vi "OSIPI OPCUA Server Tag Version.vi"(11 "Main Queue Cluster":T4) -> ()   [LabVIEW 2018]
uses:
  <vilib>/OPCUA/controls/NodeId.ctl
  <vilib>/OPCUA/controls/OPC UA Variable Node Refnum.ctl
  <vilib>/OPCUA/controls/OPC UA Server Refnum.ctl
  Drag and Drop/State Cluster.ctl
  support/Message Queue/Message Cluster.ctl
  Drag and Drop/Thumbnail Cluster.ctl
  Drag and Drop/Object Cluster.ctl
  <vilib>/Utility/miscctls.llb/LVRectTypeDef.ctl
  Drag and Drop/Object Type Enum.ctl
  <vilib>/Utility/miscctls.llb/LVPositionTypeDef.ctl
  Config Module/Controls/Main Config Cluster.ctl
  OPC Module Config.ctl
  Scale Module Folder/Measure Instrument/State Enum.ctl
  <vilib>/Utility/miscctls.llb/LVPoint32TypeDef.ctl
  OPC Settings.ctl
  Variable Data Cluster.ctl
  <vilib>/OPCUA/controls/OPC UA StatusCode.ctl
  <vilib>/OPCUA/controls/Subscription ID.ctl
  <vilib>/OPCUA/controls/OPC UA Client Refnum.ctl
  <vilib>/OPCUA/controls/Subscription Data Change.ctl
  <vilib>/OPCUA/controls/Data Type.ctl
  OPC Tag Data.ctl
  Feed Module/Controls/Feed Module Config Cluster.ctl
  Feed Module/Controls/Feed Module Settings Cluster.ctl
  Ismatec ISM 831C/Controls/Ismatech ISM831C Settings Cluster.ctl
  Masterflex 7550-30/Controls/Settings Cluster.ctl
  Mettler Toledo/Controls/Settings Cluster.ctl
  Bronkhorst M13 Flow Meter/Settings Cluster.ctl
  Measure Instrument/PID 2 Parameters Cluster.ctl
  Measure Instrument/PID Input Enum.ctl
  Measure Instrument/PID 2 Output Enum.ctl
  Tacmina QI/Tacmina QI DAQ Setting.ctl
  KNF Pump/Settings Cluster plus SIMDOS.ctl
  ASIA Pump/Pump Settings.ctl
  VICI M50 Party Mode/Settings Cluster.ctl
  FLOM Pump/Settings Cluster.ctl
  SSI PR Class/SSI PR or LD Settings Cluster.ctl
  Masterflex 75211/Masterflex 75211 DAQ Setting.ctl
  SSI PR Class/SSI P40 Settings Cluster.ctl
  Ismatec 78001/Ismatec 4083.ctl
  Bronkhorst M14 Flow Meter/Settings Cluster.ctl
  TT Module/Controls/TT Module Config Cluster.ctl
  Tag VIs/Numeric Alarm Settings Cluster.ctl
  Acquisition/Hardware Configuration.ctl
  Acquisition/Task Cluster.ctl
  PT Module/Controls/PT Module Config Cluster.ctl
  Scale Module Folder/Feed Module/Controls/Scale Module Config Cluster.ctl
  Scale Module Folder/Feed Module/Controls/Scale Module Settings Cluster.ctl
  Pump Module Folder/Pump Module Config Cluster.ctl
  Pump Module Folder/Pump Module Settings Cluster.ctl
  LabJack Module/Controls/U3 Module Config Cluster.ctl
  Decoration Module/Decoration Module Config Cluster.ctl
  Flow Module Folder/Feed Module/Controls/Flow Module Config Cluster.ctl
  Flow Module Folder/Feed Module/Controls/Flow Module Settings Cluster.ctl
  TCU Module/TCU Module Folder/TCU Module Config Cluster.ctl
  TCU Module/TCU Module Folder/TCU Module Settings Cluster.ctl
  TCU Module/TCU Module Folder/Measure Instrument/Output Devices.ctl
  Huber TCU/Huber Settings.ctl
  Lauda Integral XT-150 TCU/Lauda Settings.ctl
  Julabo Type 1 TCU/Julabo Type 1 TCU Folder/Julabo FP-50 Settings.ctl
  Huber Unistat 410 TCU/Huber Unistat 410 RS485 Settings.ctl
  D-O Module Folder/Not Sure Where this is Used.ctl
  Sequencing/Squence Control.ctl
  D-O Module Folder/D-O Module Config Cluster.ctl
  D-O Module Folder/Valve Clusters.ctl
  D-O Module Folder/D-O Module Settings Cluster.ctl
  D-O Module Folder/D-O Device Settings Cluster.ctl
  VICI Electronic Actuator/VICI Electronic Actuator Settings.ctl
  Pressure Regulator Control Module/Pressure Regulator/Controls/4-20mA Module Config Cluster.ctl
  Pressure Regulator Control Module/Pressure Regulator/Controls/4-20mA Module Settings Cluster.ctl
  Pressure Transmitter/Pressure Transmitter Device Settings.ctl
  Pressure Reg Module/Pressure Regulator Device Settings.ctl
  Sonicator Module Folder/Feed Module/Controls/Sonicator Module Config Cluster.ctl
  Sonicator Module Folder/Feed Module/Controls/Sonicator Module Settings Cluster.ctl
  Sonic Systems P100/Sonic Systems P100 Settings.ctl
  Agitator Module Folder/Feed Module/Controls/Agitator Module Config Cluster.ctl
  Agitator Module Folder/Feed Module/Controls/Agitator Module Settings Cluster.ctl
  <vilib>/OPCUA/controls/Supported Security Policies.ctl
  Main/Main Queue Cluster.ctl
  Tag VIs/Tag FGV Operation Enum.ctl
  <vilib>/OPCUA/server/Write Double.vi
  <vilib>/regexp/Match Regular Expression.xnode
  <vilib>/OPCUA/NI OPC UA Server.lvlib
  Shared Variables/Dynamic Shared Variables.lvlib
  support/Message Queue/Message Queue.lvlib
  support/Message Queue/Enqueue Message (Single).vi
  TT Module/TT Module.lvlib
  Masterflex 7550-30/Masterflex 7550-30.lvlib
  Ismatec ISM 831C/Ismatec ISM 831C.lvlib
  Tacmina QI/Tacmina QI.lvlib
  KNF Pump/KNF SIMDOS.lvlib
  VICI M50 Party Mode/VICI M6 M50 Party Mode.lvlib
  FLOM Pump/FLOM Pump.lvlib
  ASIA Pump.lvlib
  Mettler Toledo/Mettler Toledo.lvlib
  Bronkhorst M13 Flow Meter/Bronkhorst M13 Flow Meter.lvlib
  SSI PR Class/SSI PR or LD Pump.lvlib
  Feed Module/Feed Module.lvlib
  DAQ/DAQ.lvlib
  PT Module/PT Module.lvlib
  Scale Module Folder/Scale Module.lvlib
  Pump Module Folder/Pump Module.lvlib
  LabJack Module/U3 Module.lvlib
  Flow Module Folder/Flow Module.lvlib
  Huber TCU/Huber Ministat 230 TCU.lvlib
  Lauda Integral XT-150 TCU/Lauda TCU.lvlib
  Julabo Type 1 TCU/Julabo Type 1 TCU Folder/Julabo Type FP-50 TCU.lvlib
  TCU Module/TCU Module Folder/TCU Module.lvlib
  Sequencing/Sequencing Library.lvlib
  D-O Module Folder/D-O Module.lvlib
  D-O Module Folder/DIO Valve/VICI Electronic Actuator.lvlib
  Pressure Transmitter/Pressure Transmitter Library.lvlib
  Pressure Reg Module/Pressure Regulator Library.lvlib
  Pressure Regulator Control Module/Pressure Regulator/4-20mA Module.lvlib
  OPC UA.lvlib
  Scale Module Folder/Measure Instrument/Scale Module Engine.lvlib
  Config Module/Config Module.lvlib
  Drag and Drop/Drag and Drop.lvlib
  Masterflex 75211/Masterflex 75211.lvlib
  SSI PR Class/SSI P40 Pump.lvlib
  Huber Unistat 410 TCU/Huber Unistat 410 TCU.lvlib
  Ismatec 78001/Ismatec 4308.lvlib
  Bronkhorst M14 Flow Meter/Bronkhorst M14 Flow Meter.lvlib
  Sonicator Module Folder/Sonicator Module.lvlib
  Sonic Systems P100/Sonic Systems P100.lvlib
  Agitator Module Folder/Agitator Module.lvlib
panel:
  out "Array 4":T3(array[cluster])
  in  "?":T5 {"Main Config"."PR Module Configs"."Settings"."PID 2 Parameters"."output range"."output low" format="%.2f"; "Main Config"."PR Module Configs"."Settings"."PID 2 Parameters"."output range"."output high" min=0.0 max=100.0 format="%.2f"; "Main Config"."PR Module Configs"."Settings"."PID 2 Parameters"."PID gains"."derivative time (Td, min)" format="%.3f"; "Main Config"."PR Module Configs"."Settings"."PID 2 Parameters"."PID gains"."integral time (Ti, min)" format="%.3f"; "Main Config"."PR Module Configs"."Settings"."PID 2 Parameters"."PID gains"."proportional gain (Kc)" format="%.3f"; "Main Config"."Steps"."Control" items=["Pump %", "Setpoint"]; "Main Config"."TCU Module Configs"."Settings"."Huber Unistat 410 Settings"."Address" min=0 max=99 format="%02.0f"; "Main Config"."TCU Module Configs"."Settings"."Julabo FP-50 Settings"."Pump Power" min=0 max=8 step=1; "Main Config"."TCU Module Configs"."Settings"."Lauda Settings"."Pump Power" min=0 max=8 step=1; "Main Config"."Flow Module Configs"."Settings"."Bronkhorst M14 Settings"."Smoothing Steps" min=1 step=1; "Main Config"."Flow Module Configs"."Settings"."Bronkhorst M13 Settings"."Smoothing Steps" min=1 step=1; "Main Config"."Pump Module Configs"."Settings"."Ismatech 3 Channel Settings"."Channel Number" min=0 max=3; "Main Config"."Pump Module Configs"."Settings"."Ismatech 3 Channel Settings"."Pump Number" min=1; "Main Config"."Pump Module Configs"."Settings"."ASIA Pump C"."channel" min=0 max=1 step=1; "Main Config"."Pump Module Configs"."Settings"."Masterflex"."Pump Number" min=1.0 max=20.0 step=1.0; "Main Config"."Pump Module Configs"."Settings"."Ismatech"."Pump Number" min=1.0 max=20.0 step=1.0; "Main Config"."Feed Module Configs"."Settings"."Bronkhorst M14 Settings"."Smoothing Steps" min=1 step=1; "Main Config"."Feed Module Configs"."Settings"."Ismatech 3 Channel Settings"."Channel Number" min=0 max=3; "Main Config"."Feed Module Configs"."Settings"."Ismatech 3 Channel Settings"."Pump Number" min=1; "Main Config"."Feed Module Configs"."Settings"."output range"."output low" min=0.0 max=100.0 format="%.2f"; "Main Config"."Feed Module Configs"."Settings"."output range"."output high" format="%.2f"; "Main Config"."Feed Module Configs"."Settings"."PID 2 Parameters"."PID gains"."derivative time (Td, min)" format="%.3f"; "Main Config"."Feed Module Configs"."Settings"."PID 2 Parameters"."PID gains"."integral time (Ti, min)" format="%.3f"; "Main Config"."Feed Module Configs"."Settings"."PID 2 Parameters"."PID gains"."proportional gain (Kc)" format="%.3f"; "Main Config"."Feed Module Configs"."Settings"."Bronkhorst M13 Flow Meter"."Smoothing Steps" min=1 step=1; "Main Config"."Feed Module Configs"."Settings"."ASIA Pump C"."channel" min=0 max=1 step=1; "Main Config"."Feed Module Configs"."Settings"."Ismatech"."Pump Number" min=1.0 max=20.0 step=1.0; "Main Config"."Feed Module Configs"."Settings"."Masterflex"."Pump Number" min=1.0 max=20.0 step=1.0}
  in  "supported security policies (None)":T76={"None"=TRUE, "Sign with Basic128Rsa15"=TRUE, "Sign and Encrypt with Basic128Rsa15"=TRUE, "Sign with Basic256"=TRUE, "Sign and Encrypt with Basic256"=TRUE}
  out "Tag Values":dbl[](array[numeric])
  out "Tag Names":string[](array[string])
  out "Array":T3(array[cluster])
  out "OPC UA server refnum out":T77
  out "Array 2":T17[](array[typedef]) items=["Good"=0, "Good_SubscriptionTransferred"=2949120, "Good_CompletesAsynchronously"=3014656, "Good_Overload"=3080192, "Good_Clamped"=3145728, "Good_LocalOverride"=9830400, "Good_EntryInserted"=10616832, "Good_EntryReplaced"=10682368, "Good_NoData"=10813440, "Good_MoreData"=10878976, "Good_CommunicationEvent"=10944512, "Good_ShutdownEvent"=11010048, "Good_CallAgain"=11075584, "Good_NonCriticalTimeout"=11141120, "Good_ResultsMayBeIncomplete"=12189696, "Good_DataIgnored"=14221312, "Uncertain"=1073741824, "Uncertain_ReferenceOutOfServer"=1080819712, "Uncertain_NoCommunicationLastUsableValue"=1083113472, "Uncertain_LastUsableValue"=1083179008, "Uncertain_SubstituteValue"=1083244544, "Uncertain_InitialValue"=1083310080, "Uncertain_SensorNotAccurate"=1083375616, "Uncertain_EngineeringUnitsExceeded"=1083441152, "Uncertain_SubNormal"=1083506688, "Uncertain_DataSubNormal"=1084489728, "Uncertain_ReferenceNotDeleted"=1086062592, "Uncertain_NotAllNodesAvailable"=1086324736, "Bad"=2147483648, "Bad_UnexpectedError"=2147549184, "Bad_InternalError"=2147614720, "Bad_OutOfMemory"=2147680256, "Bad_ResourceUnavailable"=2147745792, "Bad_CommunicationError"=2147811328, "Bad_EncodingError"=2147876864, "Bad_DecodingError"=2147942400, "Bad_EncodingLimitsExceeded"=2148007936, "Bad_UnknownResponse"=2148073472, "Bad_Timeout"=2148139008, "Bad_ServiceUnsupported"=2148204544, "Bad_Shutdown"=2148270080, "Bad_ServerNotConnected"=2148335616, "Bad_ServerHalted"=2148401152, "Bad_NothingToDo"=2148466688, "Bad_TooManyOperations"=2148532224, "Bad_DataTypeIdUnknown"=2148597760, "Bad_CertificateInvalid"=2148663296, "Bad_SecurityChecksFailed"=2148728832, "Bad_CertificateTimeInvalid"=2148794368, "Bad_CertificateIssuerTimeInvalid"=2148859904, "Bad_CertificateHostNameInvalid"=2148925440, "Bad_CertificateUriInvalid"=2148990976, "Bad_CertificateUseNotAllowed"=2149056512, "Bad_CertificateIssuerUseNotAllowed"=2149122048, "Bad_CertificateUntrusted"=2149187584, "Bad_CertificateRevocationUnknown"=2149253120, "Bad_CertificateIssuerRevocationUnknown"=2149318656, "Bad_CertificateRevoked"=2149384192, "Bad_CertificateIssuerRevoked"=2149449728, "Bad_UserAccessDenied"=2149515264, "Bad_IdentityTokenInvalid"=2149580800, "Bad_IdentityTokenRejected"=2149646336, "Bad_SecureChannelIdInvalid"=2149711872, "Bad_InvalidTimestamp"=2149777408, "Bad_NonceInvalid"=2149842944, "Bad_SessionIdInvalid"=2149908480, "Bad_SessionClosed"=2149974016, "Bad_SessionNotActivated"=2150039552, "Bad_SubscriptionIdInvalid"=2150105088, "Bad_RequestHeaderInvalid"=2150236160, "Bad_TimestampsToReturnInvalid"=2150301696, "Bad_RequestCancelledByClient"=2150367232, "Bad_NoCommunication"=2150694912, "Bad_WaitingForInitialData"=2150760448, "Bad_NodeIdInvalid"=2150825984, "Bad_NodeIdUnknown"=2150891520, "Bad_AttributeIdInvalid"=2150957056, "Bad_IndexRangeInvalid"=2151022592, "Bad_IndexRangeNoData"=2151088128, "Bad_DataEncodingInvalid"=2151153664, "Bad_DataEncodingUnsupported"=2151219200, "Bad_NotReadable"=2151284736, "Bad_NotWritable"=2151350272, "Bad_OutOfRange"=2151415808, "Bad_NotSupported"=2151481344, "Bad_NotFound"=2151546880, "Bad_ObjectDeleted"=2151612416, "Bad_NotImplemented"=2151677952, "Bad_MonitoringModeInvalid"=2151743488, "Bad_MonitoredItemIdInvalid"=2151809024, "Bad_MonitoredItemFilterInvalid"=2151874560, "Bad_MonitoredItemFilterUnsupported"=2151940096, "Bad_FilterNotAllowed"=2152005632, "Bad_StructureMissing"=2152071168, "Bad_EventFilterInvalid"=2152136704, "Bad_ContentFilterInvalid"=2152202240, "Bad_FilterOperandInvalid"=2152267776, "Bad_ContinuationPointInvalid"=2152333312, "Bad_NoContinuationPoints"=2152398848, "Bad_ReferenceTypeIdInvalid"=2152464384, "Bad_BrowseDirectionInvalid"=2152529920, "Bad_NodeNotInView"=2152595456, "Bad_ServerUriInvalid"=2152660992, "Bad_ServerNameMissing"=2152726528, "Bad_DiscoveryUrlMissing"=2152792064, "Bad_SempahoreFileMissing"=2152857600, "Bad_RequestTypeInvalid"=2152923136, "Bad_SecurityModeRejected"=2152988672, "Bad_SecurityPolicyRejected"=2153054208, "Bad_TooManySessions"=2153119744, "Bad_UserSignatureInvalid"=2153185280, "Bad_ApplicationSignatureInvalid"=2153250816, "Bad_NoValidCertificates"=2153316352, "Bad_RequestCancelledByRequest"=2153381888, "Bad_ParentNodeIdInvalid"=2153447424, "Bad_ReferenceNotAllowed"=2153512960, "Bad_NodeIdRejected"=2153578496, "Bad_NodeIdExists"=2153644032, "Bad_NodeClassInvalid"=2153709568, "Bad_BrowseNameInvalid"=2153775104, "Bad_BrowseNameDuplicated"=2153840640, "Bad_NodeAttributesInvalid"=2153906176, "Bad_TypeDefinitionInvalid"=2153971712, "Bad_SourceNodeIdInvalid"=2154037248, "Bad_TargetNodeIdInvalid"=2154102784, "Bad_DuplicateReferenceNotAllowed"=2154168320, "Bad_InvalidSelfReference"=2154233856, "Bad_ReferenceLocalOnly"=2154299392, "Bad_NoDeleteRights"=2154364928, "Bad_ServerIndexInvalid"=2154430464, "Bad_ViewIdUnknown"=2154496000, "Bad_TooManyMatches"=2154627072, "Bad_QueryTooComplex"=2154692608, "Bad_NoMatch"=2154758144, "Bad_MaxAgeInvalid"=2154823680, "Bad_HistoryOperationInvalid"=2154889216, "Bad_HistoryOperationUnsupported"=2154954752, "Bad_WriteNotSupported"=2155020288, "Bad_TypeMismatch"=2155085824, "Bad_MethodInvalid"=2155151360, "Bad_ArgumentsMissing"=2155216896, "Bad_TooManySubscriptions"=2155282432, "Bad_TooManyPublishRequests"=2155347968, "Bad_NoSubscription"=2155413504, "Bad_SequenceNumberUnknown"=2155479040, "Bad_MessageNotAvailable"=2155544576, "Bad_InsufficientClientProfile"=2155610112, "Bad_TcpServerTooBusy"=2155675648, "Bad_TcpMessageTypeInvalid"=2155741184, "Bad_TcpSecureChannelUnknown"=2155806720, "Bad_TcpMessageTooLarge"=2155872256, "Bad_TcpNotEnoughResources"=2155937792, "Bad_TcpInternalError"=2156003328, "Bad_TcpEndpointUrlInvalid"=2156068864, "Bad_RequestInterrupted"=2156134400, "Bad_RequestTimeout"=2156199936, "Bad_SecureChannelClosed"=2156265472, "Bad_SecureChannelTokenUnknown"=2156331008, "Bad_SequenceNumberInvalid"=2156396544, "Bad_ConfigurationError"=2156462080, "Bad_NotConnected"=2156527616, "Bad_DeviceFailure"=2156593152, "Bad_SensorFailure"=2156658688, "Bad_OutOfService"=2156724224, "Bad_DeadbandFilterInvalid"=2156789760, "Bad_RefreshInProgress"=2157379584, "Bad_ConditionAlreadyDisabled"=2157445120, "Bad_ConditionDisabled"=2157510656, "Bad_EventIdUnknown"=2157576192, "Bad_NoData"=2157641728, "Bad_DataLost"=2157772800, "Bad_DataUnavailable"=2157838336, "Bad_EntryExists"=2157903872, "Bad_NoEntryExists"=2157969408, "Bad_TimestampNotSupported"=2158034944, "Bad_InvalidArgument"=2158690304, "Bad_ConnectionRejected"=2158755840, "Bad_Disconnect"=2158821376, "Bad_ConnectionClosed"=2158886912, "Bad_InvalidState"=2158952448, "Bad_EndOfStream"=2159017984, "Bad_NoDataAvailable"=2159083520, "Bad_WaitingForResponse"=2159149056, "Bad_OperationAbandoned"=2159214592, "Bad_ExpectedStreamToBlock"=2159280128, "Bad_WouldBlock"=2159345664, "Bad_SyntaxError"=2159411200, "Bad_MaxConnectionsReached"=2159476736, "Bad_RequestTooLarge"=2159542272, "Bad_ResponseTooLarge"=2159607808, "Bad_EventNotAcknowledgeable"=2159738880, "Bad_InvalidTimestampArgument"=2159869952, "Bad_ProtocolVersionUnsupported"=2159935488, "Bad_StateNotActive"=2160001024, "Bad_FilterOperatorInvalid"=2160132096, "Bad_FilterOperatorUnsupported"=2160197632, "Bad_FilterOperandCountMismatch"=2160263168, "Bad_FilterElementInvalid"=2160328704, "Bad_FilterLiteralInvalid"=2160394240, "Bad_IdentityChangeNotSupported"=2160459776, "Bad_NotTypeDefinition"=2160590848, "Bad_ViewTimestampInvalid"=2160656384, "Bad_ViewParameterMismatch"=2160721920, "Bad_ViewVersionInvalid"=2160787456, "Bad_ConditionAlreadyEnabled"=2160852992, "Bad_DialogNotActive"=2160918528, "Bad_DialogResponseInvalid"=2160984064, "Bad_ConditionBranchAlreadyAcked"=2161049600, "Bad_ConditionBranchAlreadyConfirmed"=2161115136, "Bad_ConditionAlreadyShelved"=2161180672, "Bad_ConditionNotShelved"=2161246208, "Bad_ShelvingTimeOutOfRange"=2161311744, "Bad_AggregateListMismatch"=2161377280, "Bad_AggregateNotSupported"=2161442816, "Bad_AggregateInvalidInputs"=2161508352, "Bad_BoundNotFound"=2161573888, "Bad_BoundNotSupported"=2161639424, "Bad_AggregateConfigurationRejected"=2161770496, "Bad_TooManyMonitoredItems"=2161836032]
  out "server endpoint URL":string
  in  "?":T5 {"Main Config"."PR Module Configs"."Settings"."PID 2 Parameters"."output range"."output low" format="%.2f"; "Main Config"."PR Module Configs"."Settings"."PID 2 Parameters"."output range"."output high" min=0.0 max=100.0 format="%.2f"; "Main Config"."PR Module Configs"."Settings"."PID 2 Parameters"."PID gains"."derivative time (Td, min)" format="%.3f"; "Main Config"."PR Module Configs"."Settings"."PID 2 Parameters"."PID gains"."integral time (Ti, min)" format="%.3f"; "Main Config"."PR Module Configs"."Settings"."PID 2 Parameters"."PID gains"."proportional gain (Kc)" format="%.3f"; "Main Config"."Steps"."Control" items=["Pump %", "Setpoint"]; "Main Config"."TCU Module Configs"."Settings"."Huber Unistat 410 Settings"."Address" min=0 max=99 format="%02.0f"; "Main Config"."TCU Module Configs"."Settings"."Julabo FP-50 Settings"."Pump Power" min=0 max=8 step=1; "Main Config"."TCU Module Configs"."Settings"."Lauda Settings"."Pump Power" min=0 max=8 step=1; "Main Config"."Flow Module Configs"."Settings"."Bronkhorst M14 Settings"."Smoothing Steps" min=1 step=1; "Main Config"."Flow Module Configs"."Settings"."Bronkhorst M13 Settings"."Smoothing Steps" min=1 step=1; "Main Config"."Pump Module Configs"."Settings"."Ismatech 3 Channel Settings"."Channel Number" min=0 max=3; "Main Config"."Pump Module Configs"."Settings"."Ismatech 3 Channel Settings"."Pump Number" min=1; "Main Config"."Pump Module Configs"."Settings"."ASIA Pump C"."channel" min=0 max=1 step=1; "Main Config"."Pump Module Configs"."Settings"."Masterflex"."Pump Number" min=1.0 max=20.0 step=1.0; "Main Config"."Pump Module Configs"."Settings"."Ismatech"."Pump Number" min=1.0 max=20.0 step=1.0; "Main Config"."Feed Module Configs"."Settings"."Bronkhorst M14 Settings"."Smoothing Steps" min=1 step=1; "Main Config"."Feed Module Configs"."Settings"."Ismatech 3 Channel Settings"."Channel Number" min=0 max=3; "Main Config"."Feed Module Configs"."Settings"."Ismatech 3 Channel Settings"."Pump Number" min=1; "Main Config"."Feed Module Configs"."Settings"."output range"."output low" min=0.0 max=100.0 format="%.2f"; "Main Config"."Feed Module Configs"."Settings"."output range"."output high" format="%.2f"; "Main Config"."Feed Module Configs"."Settings"."PID 2 Parameters"."PID gains"."derivative time (Td, min)" format="%.3f"; "Main Config"."Feed Module Configs"."Settings"."PID 2 Parameters"."PID gains"."integral time (Ti, min)" format="%.3f"; "Main Config"."Feed Module Configs"."Settings"."PID 2 Parameters"."PID gains"."proportional gain (Kc)" format="%.3f"; "Main Config"."Feed Module Configs"."Settings"."Bronkhorst M13 Flow Meter"."Smoothing Steps" min=1 step=1; "Main Config"."Feed Module Configs"."Settings"."ASIA Pump C"."channel" min=0 max=1 step=1; "Main Config"."Feed Module Configs"."Settings"."Ismatech"."Pump Number" min=1.0 max=20.0 step=1.0; "Main Config"."Feed Module Configs"."Settings"."Masterflex"."Pump Number" min=1.0 max=20.0 step=1.0}
  out "OPC UA server refnum out 3":T77
  out "Array 3":T3(array[cluster])
  # "Agitator Settings"
  # "Sonicator Settings"
  # "Instrument Settings"
  # "Instrument Settings"
  # "Output Instruments"
  # "Flow Meter Settings"
  # "Output Instruments"
  # "Scale Settings"
  # "Output Instruments"
  # "Input Instruments"
  # "Agitator Settings"
  # "Sonicator Settings"
  # "Instrument Settings"
  # "Instrument Settings"
  # "Output Instruments"
  # "Flow Meter Settings"
  # "Output Instruments"
  # "Scale Settings"
  # "Output Instruments"
  # "Input Instruments"
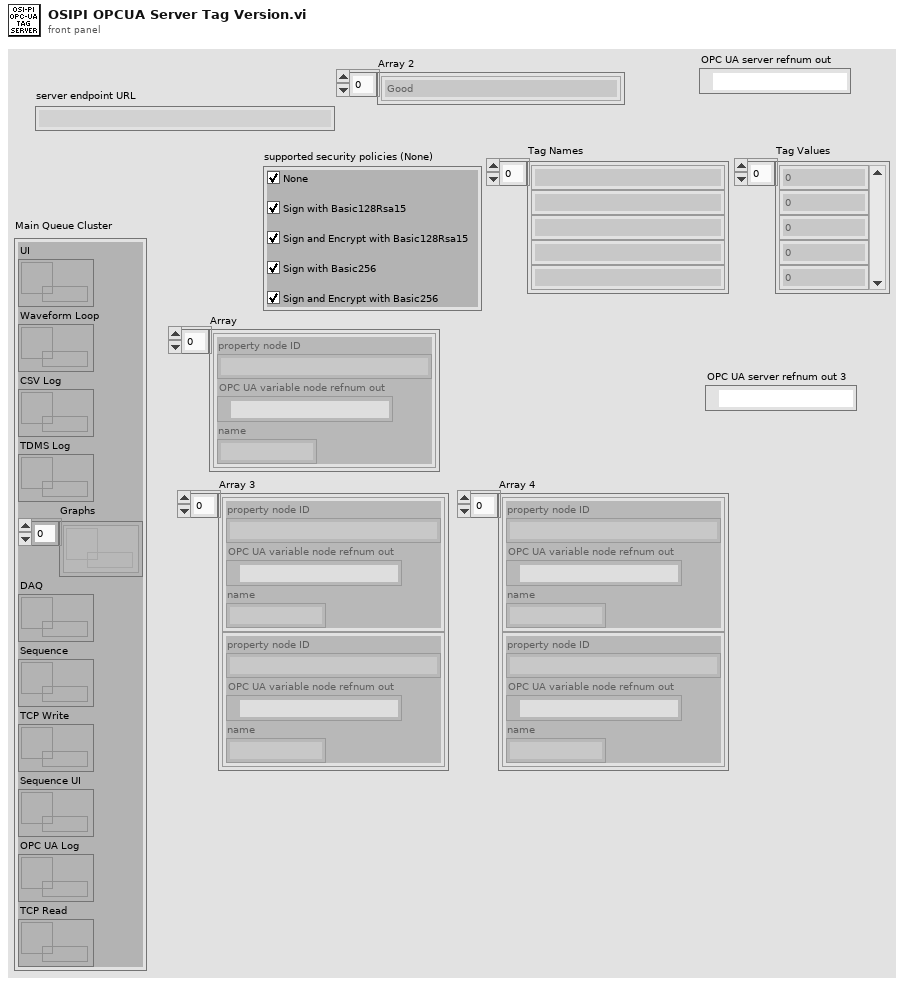
[diagram p1: front panel]
types:
  T1 = typedef "NodeId.ctl" = string
  T2 = typedef "OPC UA Variable Node Refnum.ctl" = refnum<k21>
  T3 = cluster{"property node ID":T1, "OPC UA variable node refnum out":T2, "name":string}[]
  T4 = typedef "Main Queue Cluster.ctl" = cluster{"UI":refnum<queue>, "Waveform Loop":refnum<queue>, "CSV Log":refnum<queue>, "TDMS Log":refnum<queue>, "Graphs":refnum<queue>[], "DAQ":refnum<queue>, "Sequence":refnum<queue>, "TCP Write":refnum<queue>, "Sequence UI":refnum<queue>, "OPC UA Log":refnum<queue>, "TCP Read":refnum<queue>}
  T5 = typedef "Drag and Drop.lvlib/State Cluster.ctl" = cluster{"VI refs":refnum<vi>[], "Queues":refnum<queue>[], "[Thumbnails]":T6[], "Drag Object Idx":i32, "[Objects]":T7[], "Active Object":i32, "Drop Offset":T10, "Process Name":string, "Main Config":T11, "Campaign Filepath":path, "Config Changed?":bool}
  T6 = typedef "Thumbnail Cluster.ctl" = cluster{"Path":path, "Rectangle":cluster{"left":i16, "top":i16, "right":i16, "bottom":i16}}
  T7 = typedef "Object Cluster.ctl" = cluster{"BMP Path":path, "Anchor Position":cluster{"X":i32, "Y":i32}, "Hot Spot":T8, "Type":T9, "Parameters":variant}
  T8 = typedef "LVRectTypeDef.ctl" = cluster{"Left":i16, "Top":i16, "Right":i16, "Bottom":i16}
  T9 = typedef "Object Type Enum.ctl" = enum16{"Icon", "Line", "Text", "Feed Module"}
  T10 = typedef "LVPositionTypeDef.ctl" = cluster{"Left":i32, "Top":i32}
  T11 = typedef "Config Module.lvlib/Main Config Cluster.ctl" = cluster{"Notebook":string, "OPC Module Configs":T12[], "Feed Module Configs":T21[], "Log File Path":path, "TT Module Configs":T40[], "DAQ Config":T42, "PT Module Configs":T44[], "Scale Module Configs":T45[], "Pump Module Configs":T47[], "U3 Module Configs":T49[], "Decoration Module Configs":T50[], "Flow Module Configs":T51[], "TCU Module Configs":T53[], "Steps":T60, "Abort":bool, "DO Module Configs":T62[], "PR Module Configs":T67[], "SC Module Configs":T71[], "AM Module Configs":T74[], "Cycle Period":dbl}
  T12 = typedef "OPC UA.lvlib/OPC Module Config.ctl" = cluster{"State":T13, "GUID":string, "Drop Coords":T14, "Configuration":T15, "First Iteration":bool, "Data":cluster{"Object Name":string, "Variable Array":T16[]}[], "Process Name":string, "Load Count":i32, "Log Started":bool, "subscription ID out":T18, "OPC UA client refnum out":T19, "Event Registration Refnum":refnum<event-registration>, "Start Time":timestamp, "Current Time":timestamp, "Tag Data":T20[]}
  T13 = typedef "Scale Module.lvlib/Scale Module Engine.lvlib/State Enum.ctl" = enum16{"Measuring", "Idle"}
  T14 = typedef "LVPoint32TypeDef.ctl" = cluster{"Horizontal":i32, "Vertical":i32}
  T15 = typedef "OPC UA.lvlib/OPC Settings.ctl" = cluster{"Cycle Period":dbl, "server endpoint URL":string, "security policy":cluster{"message mode":enum16{"None", "Sign", "Sign and Encrypt"}, "security":enum16{"Basic256", "Basic128Rsa15"}}, "Trust Any Server":bool}
  T16 = typedef "OPC UA.lvlib/Variable Data Cluster.ctl" = cluster{"node ID":T1, "browse name":string, "status":T17, "timestamp":timestamp, "value ":variant}
  T17 = typedef "OPC UA StatusCode.ctl" = u32
  T18 = typedef "Subscription ID.ctl" = u32
  T19 = typedef "OPC UA Client Refnum.ctl" = refnum<k21>
  T20 = typedef "OPC UA.lvlib/OPC Tag Data.ctl" = cluster{"Include this Device":bool, "Device Name":string, "OPC Tag Data":cluster{"Tag":string, "Value":variant, "Time Stamp":timestamp}[]}
  T21 = typedef "Feed Module.lvlib/Feed Module Config Cluster.ctl" = cluster{"GUID":string, "Drop Coords":T14, "Process Name":string, "Queue Name":string, "Settings":T22, "Settings Load Count":i32, "OP Load Count":i32}
  T22 = typedef "Feed Module.lvlib/Feed Module Settings Cluster.ctl" = cluster{"Cycle Period":dbl, "Ismatech":T23, "Masterflex":T24, "Mettler":T25, "Bronkhorst M13 Flow Meter":T26, "PID 2 Parameters":T27, "Manual Entry":dbl, "Auto?":bool, "output range":cluster{"output high":dbl, "output low":dbl}, "Tacmina Settings":T30, "KNF SIMDOS Settings":T31, "ASIA Pump C":T32, "VICI Settings":T33, "FLOM Settings":T34, "SSI PR/LD Settings":T35, "Masterflex 75211 Settings":T36, "SSI P40 Settings":T37, "Ismatech 3 Channel Settings":T38, "Bronkhorst M14 Settings":T39}
  T23 = typedef "Ismatec ISM 831C.lvlib/Ismatech ISM831C Settings Cluster.ctl" = cluster{"VISA resource name":refnum<visa-resource-name>, "Simulated?":bool, "Pump Number":dbl, "Reverse?":bool}
  T24 = typedef "Masterflex 7550-30.lvlib/Settings Cluster.ctl" = cluster{"VISA resource name":refnum<visa-resource-name>, "Simulated?":bool, "Pump Number":dbl, "Reverse?":bool}
  T25 = typedef "Mettler Toledo.lvlib/Settings Cluster.ctl" = cluster{"VISA resource name":refnum<visa-resource-name>, "Simulated?":bool}
  T26 = typedef "Bronkhorst M13 Flow Meter.lvlib/Settings Cluster.ctl" = cluster{"VISA resource name":refnum<visa-resource-name>, "Simulated?":bool, "Smoothing Steps":i32}
  T27 = typedef "PID 2 Parameters Cluster.ctl" = cluster{"Input Device":T28, "Output Device":T29, "Setpoint":dbl, "PID gains":cluster{"proportional gain (Kc)":dbl, "integral time (Ti, min)":dbl, "derivative time (Td, min)":dbl}}
  T28 = typedef "PID Input Enum.ctl" = enum16{"Default", "Bronkhorst M13", "Bronkhorst M14", "Scale Rate of Change"}
  T29 = typedef "PID 2 Output Enum.ctl" = enum16{"Default", "Ismatec ISM 4308", "Ismatec ISM 831C", "Masterflex 7550-30", "VICI", "Tacmina QI", "KNF SIMDOS", "ASIA Type C", "FLOM UI-22-11", "SSI PR/LD", "SSI P40", "Masterflex 75211-70"}
  T30 = typedef "Tacmina QI.lvlib/Tacmina QI DAQ Setting.ctl" = cluster{"Analog DAQ Task":refnum<k21>, "Digital DAQ Task":refnum<k21>}
  T31 = typedef "KNF SIMDOS.lvlib/Settings Cluster plus SIMDOS.ctl" = cluster{"VISA resource name":refnum<visa-resource-name>, "Simulated?":bool}
  T32 = typedef "ASIA Pump.lvlib/Pump Settings.ctl" = cluster{"ASIA Pump #":i32, "channel":i32, "Simulated":bool}
  T33 = typedef "VICI M6 M50 Party Mode.lvlib/Settings Cluster.ctl" = cluster{"VISA resource name":refnum<visa-resource-name>, "Simulated?":bool, "Pump Letter":string, "Reverse?":bool}
  T34 = typedef "FLOM Pump.lvlib/Settings Cluster.ctl" = cluster{"VISA resource name":refnum<visa-resource-name>, "Simulated?":bool, "Pump Number":dbl}
  T35 = typedef "SSI PR or LD Pump.lvlib/SSI PR or LD Settings Cluster.ctl" = cluster{"VISA resource name":refnum<visa-resource-name>, "Simulated?":bool}
  T36 = typedef "Masterflex 75211.lvlib/Masterflex 75211 DAQ Setting.ctl" = cluster{"Analog DAQ Task":refnum<k21>, "Digital DAQ Task":refnum<k21>}
  T37 = typedef "SSI P40 Pump.lvlib/SSI P40 Settings Cluster.ctl" = cluster{"VISA resource name":refnum<visa-resource-name>, "Simulated?":bool}
  T38 = typedef "Ismatec 4308.lvlib/Ismatec 4083.ctl" = cluster{"VISA resource name":refnum<visa-resource-name>, "Pump Number":i16, "Channel Number":i16, "Simulated?":bool, "Reverse?":bool}
  T39 = typedef "Bronkhorst M14 Flow Meter.lvlib/Settings Cluster.ctl" = cluster{"VISA resource name":refnum<visa-resource-name>, "Simulated?":bool, "Smoothing Steps":i32}
  T40 = typedef "TT Module.lvlib/TT Module Config Cluster.ctl" = cluster{"GUID":string, "Drop Coords":T14, "Input Channel Tag Name ":string, "Process Name":string, "Queue Name":string, "Input Channel Numeric Alarm Settings":T41[]}
  T41 = typedef "Numeric Alarm Settings Cluster.ctl" = cluster{"enable? (F)":bool, "name":string, "alarm type":enum16{"HI_HI", "HI", "LO", "LO_LO"}, "level/change":dbl, "deadband/time":dbl, "alarm delay":dbl, "priority":u32, "ack type":enum16{"Auto", "User", "None", "Each Occurrence"}, "area":string, "description":string, "log? (T)":bool}
  T42 = typedef "DAQ.lvlib/Hardware Configuration.ctl" = cluster{"Tasks":T43[]}
  T43 = typedef "Task Cluster.ctl" = cluster{"DAQmx Task":refnum<k21>, "Read-Write Radio":enum32{"Read", "Write"}}
  T44 = typedef "PT Module.lvlib/PT Module Config Cluster.ctl" = cluster{"GUID":string, "Drop Coords":T14, "Input Channel Tag Name ":string, "Process Name":string, "Queue Name":string, "Input Channel Numeric Alarm Settings":T41[]}
  T45 = typedef "Scale Module.lvlib/Scale Module Config Cluster.ctl" = cluster{"GUID":string, "Drop Coords":T14, "Process Name":string, "Queue Name":string, "Settings":T46, "Load Count":i32}
  T46 = typedef "Scale Module.lvlib/Scale Module Settings Cluster.ctl" = cluster{"Cycle Period":dbl, "Mettler":T25, "Scale Type":string}
  T47 = typedef "Pump Module.lvlib/Pump Module Config Cluster.ctl" = cluster{"GUID":string, "Drop Coords":T14, "Process Name":string, "Queue Name":string, "Settings":T48, "Load Count":i32}
  T48 = typedef "Pump Module.lvlib/Pump Module Settings Cluster.ctl" = cluster{"Cycle Period":dbl, "Manual Entry":dbl, "Output Device":T29, "Ismatech":T23, "Ismatech 3 Channel Settings":T38, "Masterflex":T24, "VICI Settings":T33, "Tacmina Settings":T30, "KNF SIMDOS Settings":T31, "ASIA Pump C":T32, "FLOM Settings":T34, "SSI PR/LD Settings":T35, "SSI P40 Settings":T35, "Masterflex 75211 Settings":T36, "Pump Calibration File":path, "Calibration Slope":dbl, "Calibration Y Intercept":dbl, "Pump Cal Enum":u16}
  T49 = typedef "U3 Module.lvlib/U3 Module Config Cluster.ctl" = cluster{"GUID":string, "Drop Coords":T14, "AI Channel Number":enum16{"Default", "AI0", "AI1", "AI2", "AI3", "AI4", "AI5", "AI6", "AI7"}, "Process Name":string, "Queue Name":string, "Input Channel Numeric Alarm Settings":T41[]}
  T50 = typedef "Decoration Module Config Cluster.ctl" = cluster{"GUID":string, "Drop Coords":T14, "Decoration Filepath":path}
  T51 = typedef "Flow Module.lvlib/Flow Module Config Cluster.ctl" = cluster{"GUID":string, "Drop Coords":T14, "Process Name":string, "Queue Name":string, "Settings":T52, "Load Count":i32}
  T52 = typedef "Flow Module.lvlib/Flow Module Settings Cluster.ctl" = cluster{"Cycle Period":dbl, "Flow Meter Type":string, "Bronkhorst M13 Settings":T26, "Bronkhorst M14 Settings":T39}
  T53 = typedef "TCU Module.lvlib/TCU Module Config Cluster.ctl" = cluster{"GUID":string, "Drop Coords":T14, "Process Name":string, "Queue Name":string, "Settings":T54, "Load Count":i32, "Power Level Changed":bool}
  T54 = typedef "TCU Module.lvlib/TCU Module Settings Cluster.ctl" = cluster{"Cycle Period":dbl, "Setpoint Entry":dbl, "Output Device":T55, "Huber Ministat 230 Settings":T56, "Lauda Settings":T57, "Julabo FP-50 Settings":T58, "Internal Control?":bool, "Huber Unistat 410 Settings":T59}
  T55 = typedef "Output Devices.ctl" = enum16{"Default", "Huber Ministat 230", "Huber Unistat 410", "Lauda XT-150", "Julabo FP-50"}
  T56 = typedef "Huber Ministat 230 TCU.lvlib/Huber Settings.ctl" = cluster{"VISA resource name":refnum<visa-resource-name>, "Simulated?":bool}
  T57 = typedef "Lauda TCU.lvlib/Lauda Settings.ctl" = cluster{"VISA resource name":refnum<visa-resource-name>, "Simulated?":bool, "Pump Power":i32}
  T58 = typedef "Julabo Type FP-50 TCU.lvlib/Julabo FP-50 Settings.ctl" = cluster{"VISA resource name":refnum<visa-resource-name>, "Simulated?":bool, "Pump Power":i32}
  T59 = typedef "Huber Unistat 410 TCU.lvlib/Huber Unistat 410 RS485 Settings.ctl" = cluster{"VISA resource name":refnum<visa-resource-name>, "Address":i8, "Simulated?":bool}
  T60 = typedef "Not Sure Where this is Used.ctl" = T61[]
  T61 = typedef "Sequencing Library.lvlib/Squence Control.ctl" = cluster{"Module":string, "Control":u16, "Value":dbl, "Wait (sec)":dbl}
  T62 = typedef "D-O Module.lvlib/D-O Module Config Cluster.ctl" = cluster{"GUID":string, "Drop Coords":T14, "Process Name":string, "Queue Name":string, "Settings":T63, "Load Count":i32}
  T63 = typedef "D-O Module.lvlib/Valve Clusters.ctl" = cluster{"Valve Settings":T64, "Valve Type":enum16{"Default", "Digital Output Valve", "VICI Electronic Actuator"}, "Time On (Sec)":dbl, "Time Off (Sec)":dbl, "Run?":bool}
  T64 = typedef "D-O Module.lvlib/D-O Module Settings Cluster.ctl" = cluster{"D-O Settings":T65, "VICI Electronic Actuator":T66}
  T65 = typedef "D-O Module.lvlib/D-O Device Settings Cluster.ctl" = cluster{"DAQmx Task Name":refnum<k21>, "Output Channel":u16, "Output Channel Names":string[]}
  T66 = typedef "VICI Electronic Actuator.lvlib/VICI Electronic Actuator Settings.ctl" = cluster{"VISA resource name":refnum<visa-resource-name>, "Mode":enum16{"Two Positions With Stops", "Two Positions Without Stops", "Mutiposition"}, "Simulated":bool}
  T67 = typedef "4-20mA Module.lvlib/4-20mA Module Config Cluster.ctl" = cluster{"GUID":string, "Drop Coords":T14, "Process Name":string, "Queue Name":string, "Settings":T68, "Settings Load Count":i32}
  T68 = typedef "4-20mA Module.lvlib/4-20mA Module Settings Cluster.ctl" = cluster{"Cycle Period":dbl, "PID 2 Parameters":cluster{"Input Device":enum16{"Default", "4-20mA"}, "Output Device":enum16{"Default", "Equilibar Pressure Reg", "Flow Regulator"}, "Setpoint":dbl, "PID gains":cluster{"proportional gain (Kc)":dbl, "integral time (Ti, min)":dbl, "derivative time (Td, min)":dbl}, "output range":cluster{"output low":dbl, "output high":dbl}}, "Manual Entry":dbl, "Auto?":bool, "4-20mA Input Settings":T69, "4-20mA Out Settings":T70, "Input Channel Tag Name ":string}
  T69 = typedef "Pressure Transmitter Library.lvlib/Pressure Transmitter Device Settings.ctl" = cluster{"Input Channel ":u16}
  T70 = typedef "Pressure Regulator Library.lvlib/Pressure Regulator Device Settings.ctl" = cluster{"Output DAQ Task":refnum<k21>}
  T71 = typedef "Sonicator Module.lvlib/Sonicator Module Config Cluster.ctl" = cluster{"GUID":string, "Drop Coords":T14, "Process Name":string, "Queue Name":string, "Settings":T72, "Load Count":i32}
  T72 = typedef "Sonicator Module.lvlib/Sonicator Module Settings Cluster.ctl" = cluster{"Cycle Period":dbl, "Sonicator Type":string, "SS P100 Settings":T73, "Setpoint (µm)":dbl, "Cutoff (µm)":dbl}
  T73 = typedef "Sonic Systems P100.lvlib/Sonic Systems P100 Settings.ctl" = cluster{"VISA resource name":refnum<visa-resource-name>, "Simulated?":bool}
  T74 = typedef "Agitator Module.lvlib/Agitator Module Config Cluster.ctl" = cluster{"GUID":string, "Drop Coords":T14, "Process Name":string, "Queue Name":string, "Settings":T75, "Load Count":i32}
  T75 = typedef "Agitator Module.lvlib/Agitator Module Settings Cluster.ctl" = cluster{"Cycle Period":dbl, "Agitator Type":string, "Setpoint (µm)":dbl}
  T76 = typedef "Supported Security Policies.ctl" = cluster{"None":bool, "Sign with Basic128Rsa15":bool, "Sign and Encrypt with Basic128Rsa15":bool, "Sign with Basic256":bool, "Sign and Encrypt with Basic256":bool}
  T77 = typedef "OPC UA Server Refnum.ctl" = refnum<k21>
  T78 = cluster{"property node ID":T1, "OPC UA variable node refnum out":T2, "name":string}
  T79 = typedef "Data Type.ctl" = u16
  T80 = cluster{"name":string, "data type":T79, "access level":u16, "description":string}
  T81 = typedef "Tag FGV Operation Enum.ctl" = enum16{"Init", "Set Notification Queue", "Create Tag", "Commit", "Write Tag (Numeric)", "Write Tag (Boolean)", "Read All Tags", "Read One Tag", "Delete Tag Category", "Set Alarm Parameters (Numeric)", "Set Alarm Parameters (Boolean)", "Enable All Alarms", "Disable All Alarms", "Delete All Tags", "Read Alarms", "Ack Alarm", "Read Alarm Parameters (Numeric)", "Read Alarm Parameters (Boolean)"}
  T82 = typedef "Feed Module.lvlib/Feed Module Tag Names Cluster.ctl" = cluster{"Pump Flow Tag":string, "PID 2 Out Tag":string, "Scale Tag":string, "Density Tag":string, "FL Temp":string, "Input Device Tag":string, "Output Device Tag":string, "Pump's Flow":string, "Pump's Pressure":string, "Overpressure Tag":string}
  T83 = typedef "Pump Module.lvlib/Pump Module Tag Names Cluster.ctl" = cluster{"Pump Speed":string, "Pump Flow":string, "Pump Pressure":string, "Output Device Tag":string, "Overpressure Tag":string}
  T84 = typedef "Flow Module.lvlib/Tag Cluster.ctl" = cluster{"Flow Tag":string, "Input Disconnected":string, "Density Tag":string, "Temp Tag":string}
  T85 = typedef "TCU Module.lvlib/TCU Module Tag Names Cluster.ctl" = cluster{"TCU Temp":string, "Output Device Tag":string, "TCU Speed":string}
  T86 = typedef "4-20mA Module.lvlib/4-20mA Module Tag Names Cluster.ctl" = cluster{"4-20mA Input":string, "PID 2 Out Tag":string, "4-20mA Output":string, "Input Device Tag":string, "Output Device Tag":string}
  T87 = cluster{"Feed Module Tags Array":T82[], "DAQ Tags Array":string[], "Scale Tags Array":cluster{"Scale Value":string, "Scale Error":string}[], "Pump Module Tags Array":T83[], "Flow Module Tags Array":T84[], "TCU Module Tags Array":T85[], "PR Module Tags Array":T86[], "OPC Module Tags Array":cluster{"OPC UA Error":string, "Array of Names":string[]}[]}
  T88 = cluster{"Scale Value":string, "Scale Error":string}[]
  T89 = cluster{"OPC UA Error":string, "Array of Names":string[]}[]
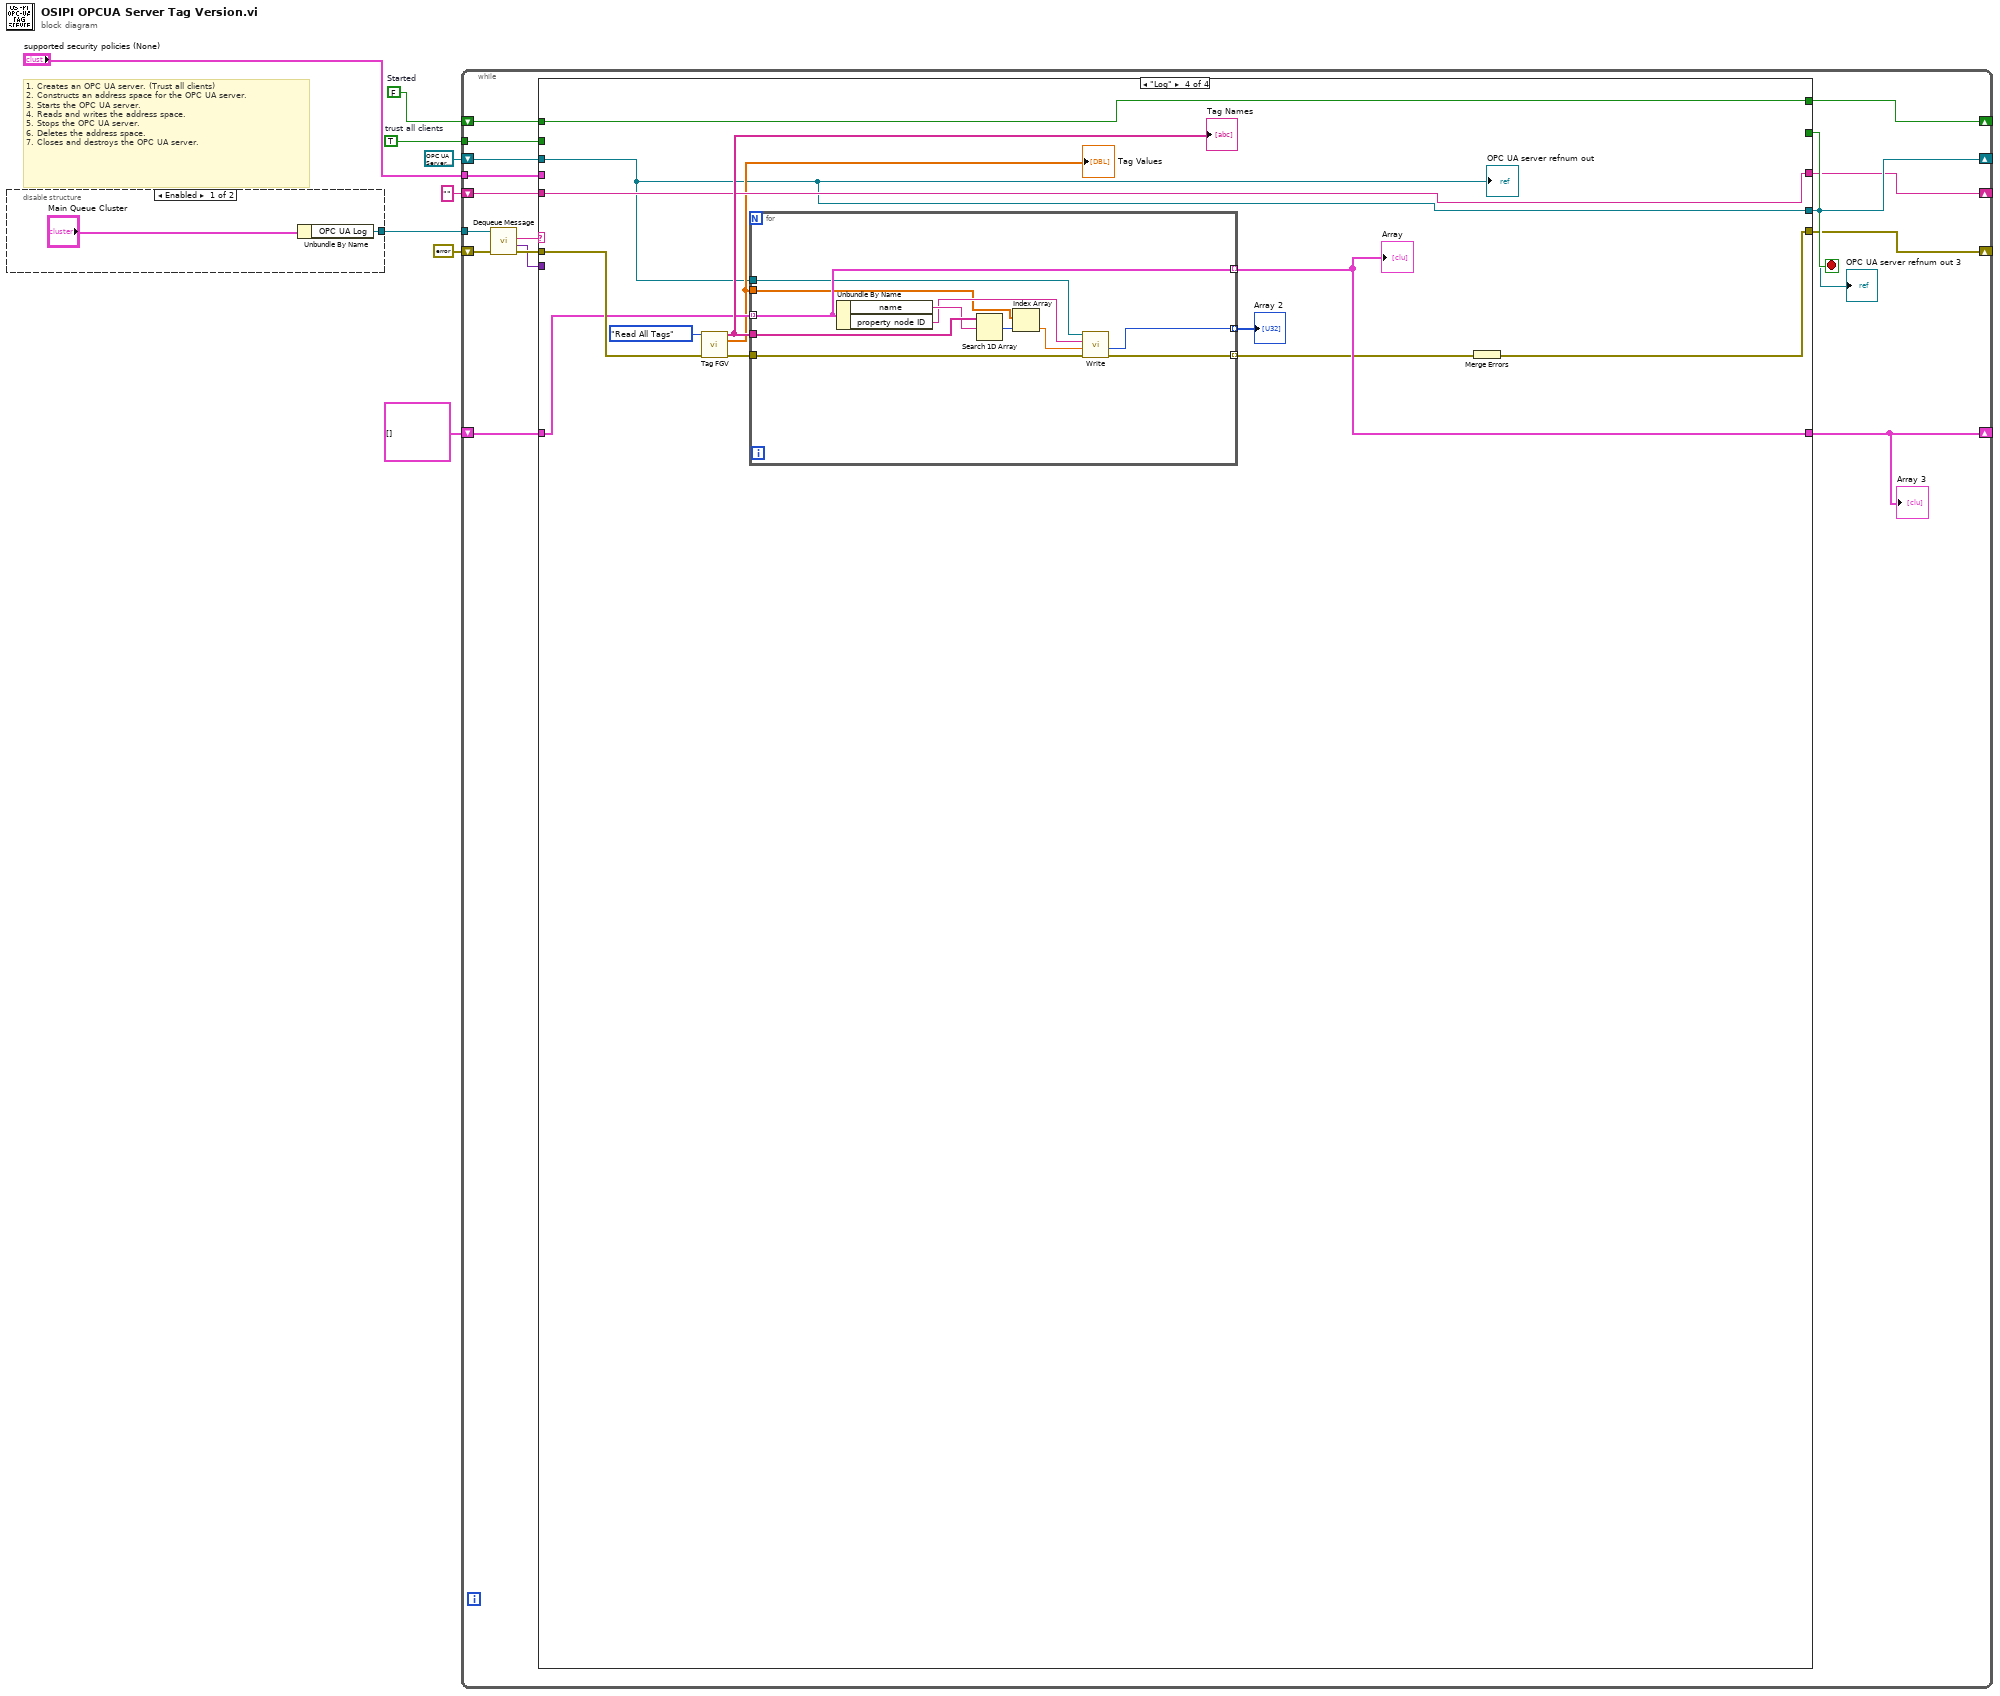
[diagram p0: block diagram]
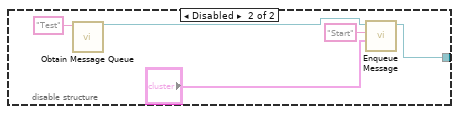
[diagram p2: hidden frame]
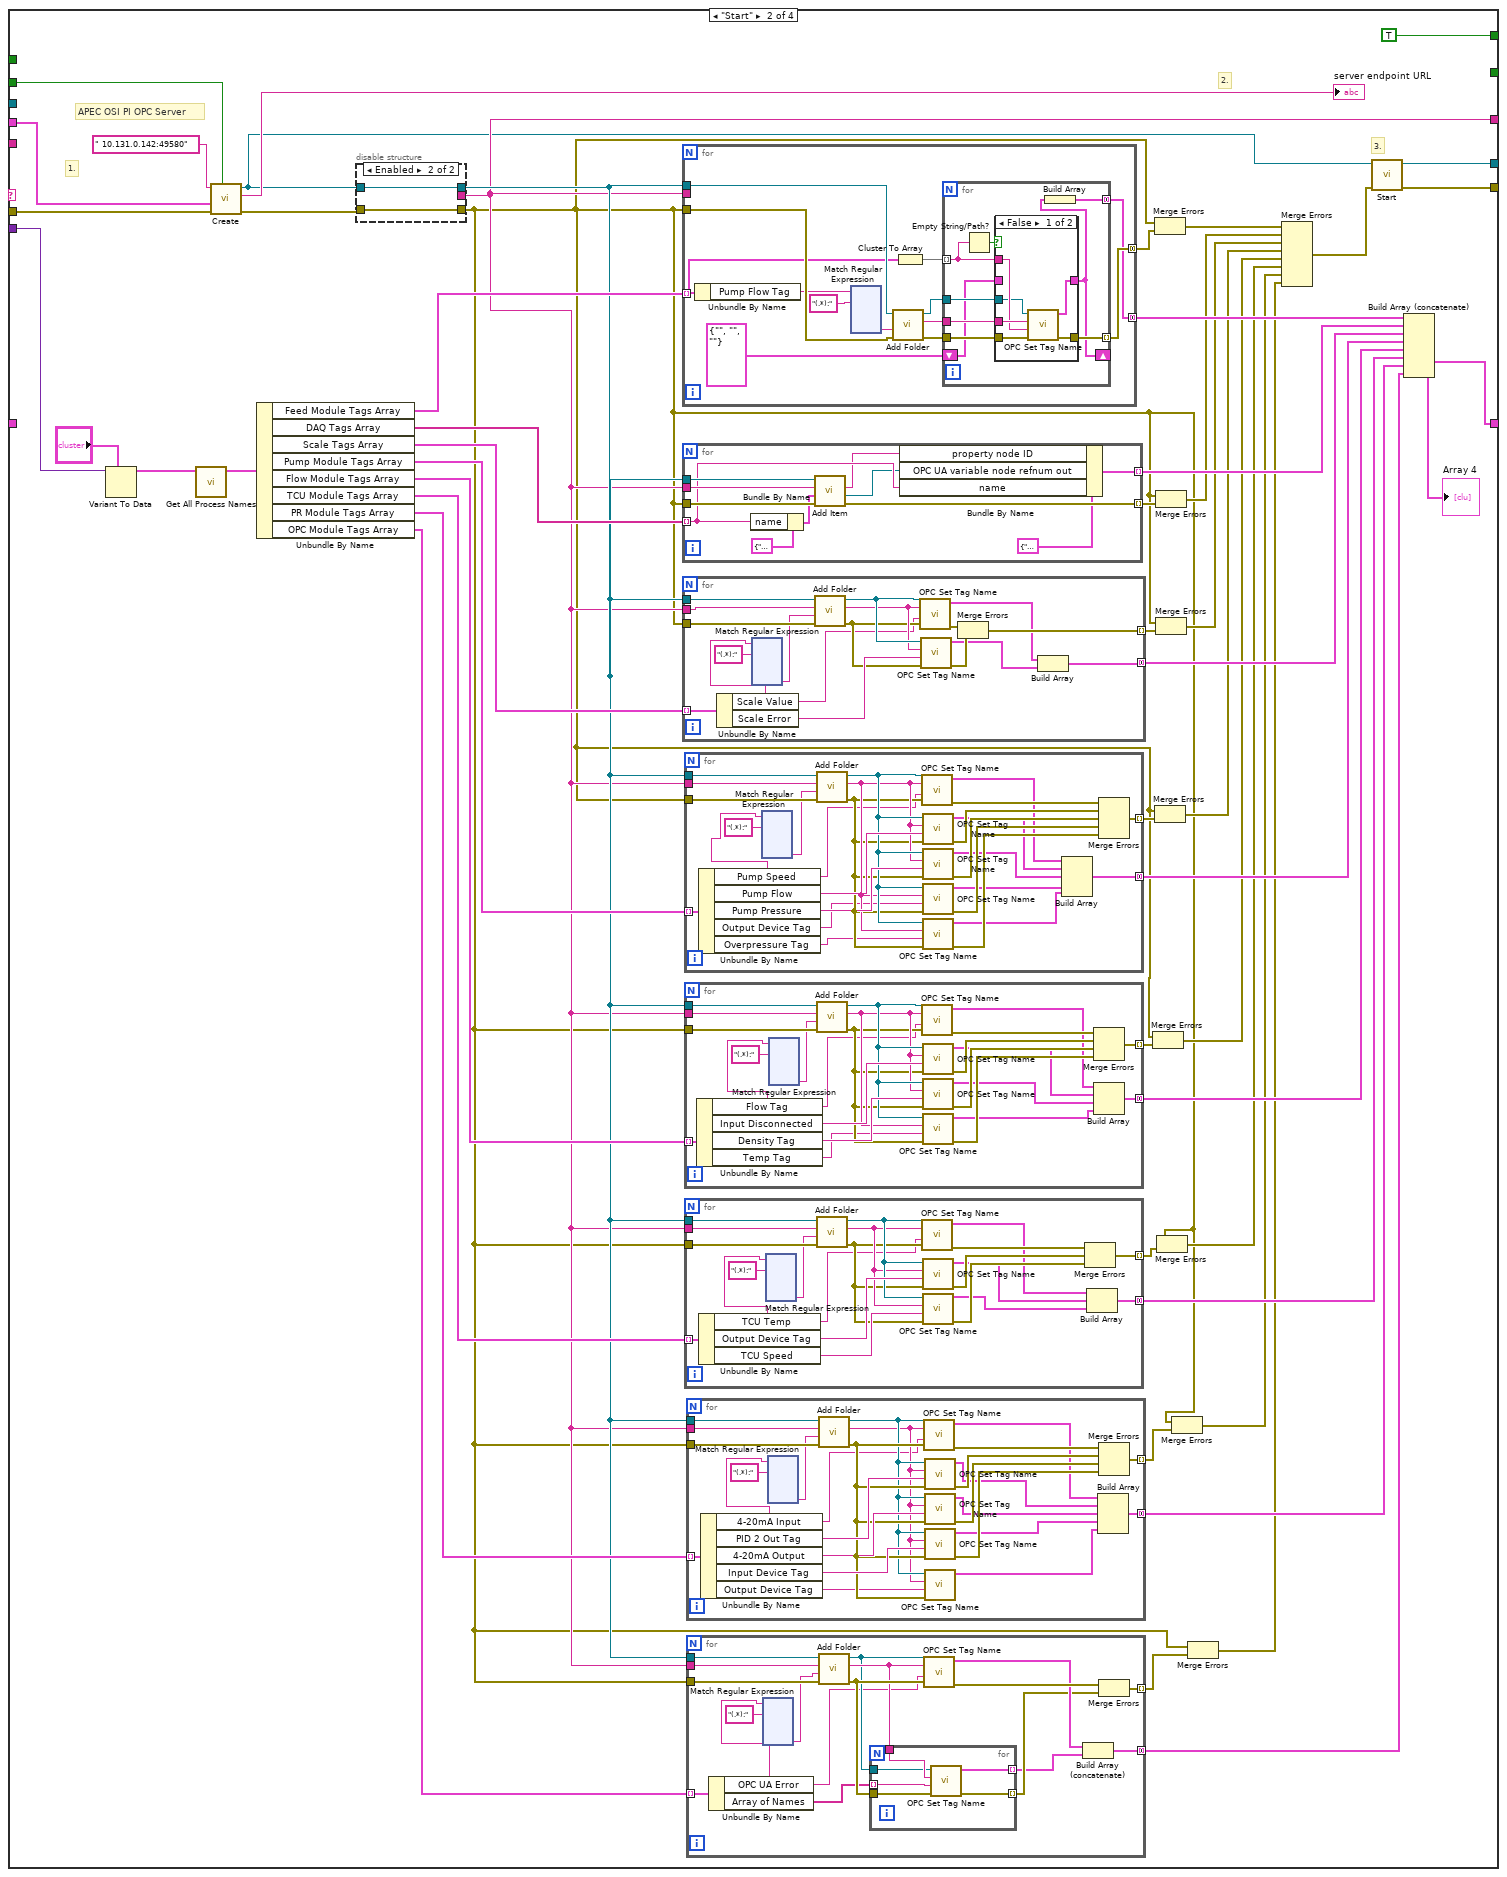
[diagram p4: hidden frame]
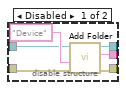
[diagram p5: hidden frame]
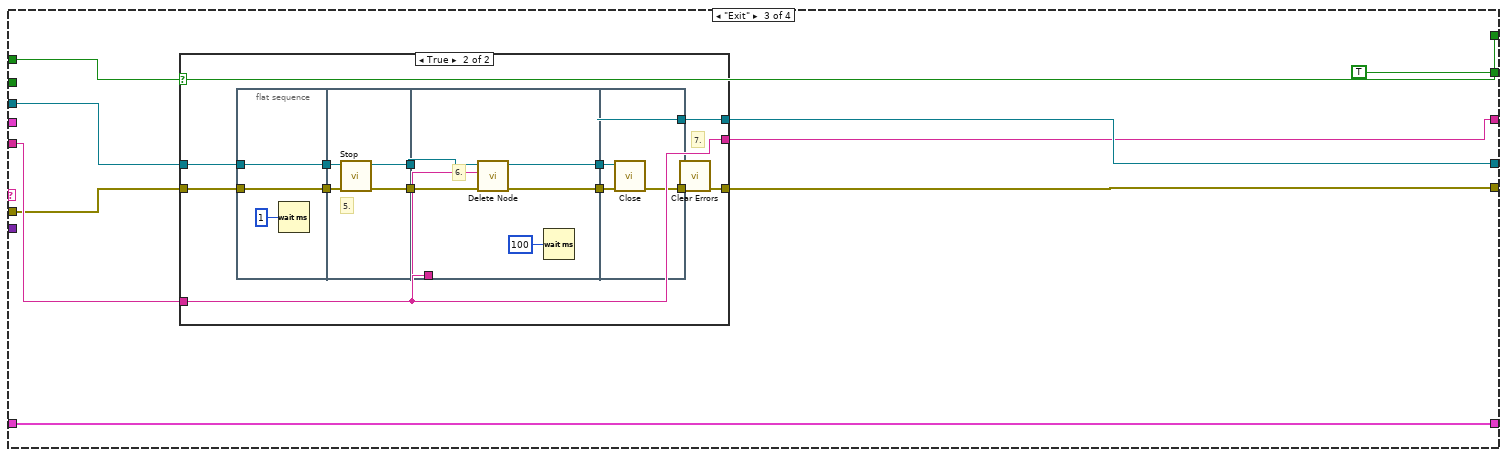
[diagram p7: hidden frame]
diagram:
  w1 = FALSE  # Started
  w8 = TRUE  # trust all clients
  # "1. Creates an OPC UA server. (Trust all clients)\n2. Constructs an address space for the OPC UA server.\n3. Starts the OPC UA server.\n4. Reads and writes the address space.\n5. Stops the OPC UA server.\n6. Deletes the address space.\n7. Closes and destroys the OPC UA server."
  n1 = disable-structure shown="Enabled" {
    disable-tunnel: [w10 w12] -> w6
    frame Enabled {
      n2 = Unbundle By Name("Main Queue Cluster") -> ("OPC UA Log"=w10:refnum<queue>)
    }
    frame Disabled {
      n3 = call "Obtain Message Queue.vi"("name (unnamed)"="Test") -> ("Message Queue"=w11:refnum<queue>)  [unwired: 9 in, 1 out]
      n4 = call-poly "Enqueue Message.vi"("Message Data"="?", "Message"="Start", "Message Queue"=w11) -> ("dup Message Queue"=w12:refnum<queue>)  [unwired: 7 in, 1 out]
    }
  }
  n5 = while {
    tunnel: w6 -> [w31]
    shift-right: [w28] -> _
    shift-left: errorcluster {"status"=FALSE, "code"=0, "source"=""} ("error IO") -> [w27]
    tunnel: w8 -> [w26]
    tunnel: "supported security policies (None)" -> [w25]
    shift-right: [w24] -> _
    shift-left: T77 refnum ("OPC UA server refnum out") -> [w23]
    shift-right: [w22] -> _
    shift-left: T1 "" ("folder node ID") -> [w20]
    shift-right: [w19] -> _
    shift-left: T3 [] -> [w18]
    shift-right: [w17] -> _
    shift-left: w1 -> [w16]
    stop <- w30 stop-if-true
    n6 = call "Dequeue Message.vi"("error in (no error)"=w27, "Message Queue"=w31) -> ("error out"=w29:errorcluster, "Message Data"=w21:variant, "Message"=w32:string)  [unwired: 6 in, 1 out]
    n7 = case shown="\"Log\"" w32 {
      tunnel: [_ _ TRUE _] -> w30
      tunnel: w29 -> [w35 w85 w1084 w1133]
      tunnel: [w35 w83 w1091 w1128] -> w28
      tunnel: w26 -> [_ w87 _ _]
      tunnel: w25 -> [_ w86 _ _]
      tunnel: [w36 w84 w1089 w1124] -> w24
      tunnel: w23 -> [w36 _ w1090 w1124]
      tunnel: [w37 w60 w1085 w1134] -> w22
      tunnel: w21 -> [_ w81 _ _]
      tunnel: w20 -> [w37 _ w1088 w1134]
      tunnel: [w34 w39 w1087 w1130] -> w19
      tunnel: w18 -> [w34 _ w1087 w1131]
      tunnel: w16 -> [w33 _ w1086 w1125]
      tunnel: [w33 TRUE ("Started") w1086 w1125] -> w17
      frame Default {
      }
      frame "Start" {
        # "APEC OSI PI OPC Server"
        # "3."
        # "2."
        # "1."
        n8 = Variant To Data(type="?", Variant=w81) -> (data=w79:T5)  [unwired: 1 in, 1 out]
        n9 = call "Get All Process Names.vi"(11:w79) -> ("Module Tags Array Cluster"=w77:T87)  [unwired: 10 in]
        n10 = call <vilib>:"Create.vi"("trust all clients (F)"=w87, "error in (no error)"=w85, "supported security policies (None)"=w86, "OPC UA server name"=" 10.131.0.142:49580") -> ("error out"=w82:errorcluster, "server endpoint URL"=→"server endpoint URL":string, "OPC UA server refnum out"=w58:T77)  [unwired: 5 in]
        n11 = Unbundle By Name(w77) -> ("Feed Module Tags Array"=w78:T82[], "DAQ Tags Array"=w76:string[], "Scale Tags Array"=w74:T88, "Pump Module Tags Array"=w73:T83[], "Flow Module Tags Array"=w72:T84[], "TCU Module Tags Array"=w71:T85[], "PR Module Tags Array"=w70:T86[], "OPC Module Tags Array"=w59:T89)
        n12 = disable-structure shown="Enabled" {
          disable-tunnel: w82 -> [w94 w95]
          disable-tunnel: [w92 w96] -> w61
          disable-tunnel: [w91 _] -> w60
          disable-tunnel: [w90 w95] -> w41
          disable-tunnel: w58 -> [w89 w96]
          frame Disabled {
            n13 = call <vilib>:"Add Folder.vi"("error in (no error)"=w94, "folder name"="Device", "OPC UA server refnum in"=w89) -> ("error out"=w90:errorcluster, "folder node ID"=w91:T1, "OPC UA server refnum out"=w92:T77)  [unwired: 5 in]
          }
          frame Enabled {
          }
        }
        n14 = for {
          tunnel: w41 -> [w950]
          tunnel: w60 -> [_]
          tunnel: w61 -> [w949]
          tunnel: [w940] -> w38 mode=concatenating
          tunnel: w78 -> [w945] mode=indexing
          tunnel: [w938] -> w69 mode=concatenating
          n15 = Unbundle By Name(w945) -> ("Pump Flow Tag"=w947:string)
          n16 = xnode "Match Regular Expression"("input string"=w947, "regular expression"="(.*):") -> ("submatch 1"=w946:string)  [unwired: 4 in, 5 out]
          n17 = call <vilib>:"Add Folder.vi"("error in (no error)"=w950, "folder name"=w946, "OPC UA server refnum in"=w949) -> ("error out"=w941:errorcluster, "folder node ID"=w943:T1, "OPC UA server refnum out"=w942:T77)  [unwired: 5 in]
          n18 = Cluster To Array(cluster=w945) -> (array=w944:string[])
          n19 = for {
            tunnel: w944 -> [w954] mode=indexing
            tunnel: w943 -> [w959]
            tunnel: w941 -> [w958]
            tunnel: w942 -> [w957]
            tunnel: [w956] -> w940 mode=indexing
            shift-right: [w952] -> _
            shift-left: T78 {"property node ID"="", "OPC UA variable node refnum out"="", "name"=""} ("OPC Property cluster") -> [w953]
            tunnel: [w951] -> w938 mode=concatenating
            n20 = Empty String/Path?(string/path=w954) -> (empty?=w955:bool)
            n21 = case shown="False" w955 {
              tunnel: w959 -> [w965 _]
              tunnel: w954 -> [w964 _]
              tunnel: w958 -> [w963 w967]
              tunnel: w957 -> [w962 _]
              tunnel: [w961 w967] -> w956
              tunnel: [w960 w966] -> w952
              tunnel: w953 -> [_ w966]
              frame False {
                n22 = call "OPC Set Tag Name.vi"("error in (no error)"=w963, "name"=w964, "item node ID"=w965, "Refnum in"=w962) -> ("error out"=w961:errorcluster, "OPC Property cluster"=w960:T78)  [unwired: 6 in]
              }
              frame True {
              }
            }
            n23 = Build Array(w952) -> (w951:T3)
          }
        }
        n24 = for {
          tunnel: w41 -> [w937]
          tunnel: w60 -> [w936]
          tunnel: w61 -> [w935]
          tunnel: [w932] -> w43 mode=indexing
          tunnel: w76 -> [w930] mode=indexing
          tunnel: [w927] -> w68 mode=indexing
          n25 = Bundle By Name(cluster=T80 {"name"="Node", "data type"=11, "access level"=3, "description"=""} ("item"), "name"=w930) -> (w933:T80)
          n26 = call <vilib>:"Add Item.vi"("error in (no error)"=w937, "item"=w933, "parent folder node ID"=w936, "OPC UA server refnum in"=w935) -> ("error out"=w932:errorcluster, "OPC UA variable node refnum out"=w929:T2, "item node ID"=w928:T1)  [unwired: 3 in, 1 out]
          n27 = Bundle By Name(cluster=T78 {"property node ID"="", "OPC UA variable node refnum out"="", "name"=""} ("OPC Property cluster"), "property node ID"=w928, "OPC UA variable node refnum out"=w929, "name"=w930) -> (w927:T78)
        }
        n28 = for {
          tunnel: [w809] -> w45 mode=indexing
          tunnel: w74 -> [w810] mode=indexing
          tunnel: w61 -> [w802]
          tunnel: w60 -> [w801]
          tunnel: w41 -> [w800]
          tunnel: [w797] -> w67 mode=concatenating
          n29 = Unbundle By Name(w810) -> ("Scale Value"=w795:string, "Scale Error"=w808:string)
          n30 = xnode "Match Regular Expression"("input string"=w795, "regular expression"="(.*):") -> ("submatch 1"=w794:string)  [unwired: 4 in, 5 out]
          n31 = call <vilib>:"Add Folder.vi"("error in (no error)"=w800, "folder name"=w794, "parent folder node ID"=w801, "OPC UA server refnum in"=w802) -> ("error out"=w803:errorcluster, "folder node ID"=w804:T1, "OPC UA server refnum out"=w805:T77)  [unwired: 4 in]
          n32 = call "OPC Set Tag Name.vi"("error in (no error)"=w803, "name"=w795, "item node ID"=w804, "Refnum in"=w805) -> ("error out"=w807:errorcluster, "OPC Property cluster"=w799:T78)  [unwired: 6 in]
          n33 = call "OPC Set Tag Name.vi"("error in (no error)"=w803, "name"=w808, "item node ID"=w804, "Refnum in"=w805) -> ("error out"=w806:errorcluster, "OPC Property cluster"=w798:T78)  [unwired: 6 in]
          n34 = Merge Errors(w807, w806) -> (w809:errorcluster)
          n35 = Build Array(w799, w798) -> (w797:T3)
        }
        n36 = for {
          tunnel: w41 -> [w677]
          tunnel: w60 -> [w676]
          tunnel: w61 -> [w675]
          tunnel: [w655] -> w47 mode=indexing
          tunnel: w73 -> [w674] mode=indexing
          tunnel: [w656] -> w66 mode=concatenating
          n37 = Unbundle By Name(w674) -> ("Pump Speed"=w653:string, "Pump Flow"=w672:string, "Pump Pressure"=w673:string, "Output Device Tag"=w665:string, "Overpressure Tag"=w664:string)
          n38 = xnode "Match Regular Expression"("input string"=w653, "regular expression"="(.*):") -> ("submatch 1"=w652:string)  [unwired: 4 in, 5 out]
          n39 = call <vilib>:"Add Folder.vi"("error in (no error)"=w677, "folder name"=w652, "parent folder node ID"=w676, "OPC UA server refnum in"=w675) -> ("error out"=w666:errorcluster, "folder node ID"=w667:T1, "OPC UA server refnum out"=w668:T77)  [unwired: 4 in]
          n40 = call "OPC Set Tag Name.vi"("error in (no error)"=w666, "name"=w653, "item node ID"=w667, "Refnum in"=w668) -> ("error out"=w671:errorcluster, "OPC Property cluster"=w661:T78)  [unwired: 6 in]
          n41 = call "OPC Set Tag Name.vi"("error in (no error)"=w666, "name"=w672, "item node ID"=w667, "Refnum in"=w668) -> ("error out"=w670:errorcluster, "OPC Property cluster"=w660:T78)  [unwired: 6 in]
          n42 = call "OPC Set Tag Name.vi"("error in (no error)"=w666, "name"=w673, "item node ID"=w667, "Refnum in"=w668) -> ("error out"=w669:errorcluster, "OPC Property cluster"=w659:T78)  [unwired: 6 in]
          n43 = call "OPC Set Tag Name.vi"("error in (no error)"=w666, "name"=w665, "item node ID"=w667, "Refnum in"=w668) -> ("error out"=w663:errorcluster, "OPC Property cluster"=w658:T78)  [unwired: 6 in]
          n44 = call "OPC Set Tag Name.vi"("error in (no error)"=w666, "name"=w664, "item node ID"=w667, "Refnum in"=w668) -> ("error out"=w662:errorcluster, "OPC Property cluster"=w657:T78)  [unwired: 6 in]
          n45 = Build Array(w661, w660, w659, w658, w657) -> (w656:T3)
          n46 = Merge Errors(w671, w670, w669, w663, w662) -> (w655:errorcluster)
        }
        n47 = for {
          tunnel: w41 -> [w535]
          tunnel: w60 -> [w534]
          tunnel: w61 -> [w533]
          tunnel: [w531] -> w49 mode=indexing
          tunnel: w72 -> [w532] mode=indexing
          tunnel: [w516] -> w65 mode=concatenating
          n48 = Unbundle By Name(w532) -> ("Flow Tag"=w514:string, "Input Disconnected"=w529:string, "Density Tag"=w530:string, "Temp Tag"=w522:string)
          n49 = xnode "Match Regular Expression"("input string"=w514, "regular expression"="(.*):") -> ("submatch 1"=w513:string)  [unwired: 4 in, 5 out]
          n50 = call <vilib>:"Add Folder.vi"("error in (no error)"=w535, "folder name"=w513, "parent folder node ID"=w534, "OPC UA server refnum in"=w533) -> ("error out"=w523:errorcluster, "folder node ID"=w524:T1, "OPC UA server refnum out"=w525:T77)  [unwired: 4 in]
          n51 = call "OPC Set Tag Name.vi"("error in (no error)"=w523, "name"=w514, "item node ID"=w524, "Refnum in"=w525) -> ("error out"=w528:errorcluster, "OPC Property cluster"=w520:T78)  [unwired: 6 in]
          n52 = call "OPC Set Tag Name.vi"("error in (no error)"=w523, "name"=w529, "item node ID"=w524, "Refnum in"=w525) -> ("error out"=w527:errorcluster, "OPC Property cluster"=w519:T78)  [unwired: 6 in]
          n53 = call "OPC Set Tag Name.vi"("error in (no error)"=w523, "name"=w530, "item node ID"=w524, "Refnum in"=w525) -> ("error out"=w526:errorcluster, "OPC Property cluster"=w518:T78)  [unwired: 6 in]
          n54 = call "OPC Set Tag Name.vi"("error in (no error)"=w523, "name"=w522, "item node ID"=w524, "Refnum in"=w525) -> ("error out"=w521:errorcluster, "OPC Property cluster"=w517:T78)  [unwired: 6 in]
          n55 = Merge Errors(w528, w527, w526, w521) -> (w531:errorcluster)
          n56 = Build Array(w520, w519, w518, w517) -> (w516:T3)
        }
        n57 = for {
          tunnel: w41 -> [w396]
          tunnel: w60 -> [w395]
          tunnel: w61 -> [w394]
          tunnel: [w392] -> w51 mode=indexing
          tunnel: w71 -> [w393] mode=indexing
          tunnel: [w380] -> w64 mode=concatenating
          n58 = Unbundle By Name(w393) -> ("TCU Temp"=w377:string, "Output Device Tag"=w390:string, "TCU Speed"=w391:string)
          n59 = xnode "Match Regular Expression"("input string"=w377, "regular expression"="(.*):") -> ("submatch 1"=w378:string)  [unwired: 4 in, 5 out]
          n60 = call <vilib>:"Add Folder.vi"("error in (no error)"=w396, "folder name"=w378, "parent folder node ID"=w395, "OPC UA server refnum in"=w394) -> ("error out"=w384:errorcluster, "folder node ID"=w385:T1, "OPC UA server refnum out"=w386:T77)  [unwired: 4 in]
          n61 = call "OPC Set Tag Name.vi"("error in (no error)"=w384, "name"=w377, "item node ID"=w385, "Refnum in"=w386) -> ("error out"=w389:errorcluster, "OPC Property cluster"=w383:T78)  [unwired: 6 in]
          n62 = call "OPC Set Tag Name.vi"("error in (no error)"=w384, "name"=w390, "item node ID"=w385, "Refnum in"=w386) -> ("error out"=w388:errorcluster, "OPC Property cluster"=w382:T78)  [unwired: 6 in]
          n63 = call "OPC Set Tag Name.vi"("error in (no error)"=w384, "name"=w391, "item node ID"=w385, "Refnum in"=w386) -> ("error out"=w387:errorcluster, "OPC Property cluster"=w381:T78)  [unwired: 6 in]
          n64 = Merge Errors(w389, w388, w387) -> (w392:errorcluster)
          n65 = Build Array(w383, w382, w381) -> (w380:T3)
        }
        n66 = for {
          tunnel: w41 -> [w260]
          tunnel: w60 -> [w259]
          tunnel: w61 -> [w258]
          tunnel: [w256] -> w53 mode=indexing
          tunnel: w70 -> [w257] mode=indexing
          tunnel: [w239] -> w63 mode=concatenating
          n67 = Unbundle By Name(w257) -> ("4-20mA Input"=w237:string, "PID 2 Out Tag"=w254:string, "4-20mA Output"=w255:string, "Input Device Tag"=w249:string, "Output Device Tag"=w245:string)
          n68 = xnode "Match Regular Expression"("input string"=w237, "regular expression"="(.*):") -> ("submatch 1"=w236:string)  [unwired: 4 in, 5 out]
          n69 = call <vilib>:"Add Folder.vi"("error in (no error)"=w260, "folder name"=w236, "parent folder node ID"=w259, "OPC UA server refnum in"=w258) -> ("error out"=w248:errorcluster, "folder node ID"=w246:T1, "OPC UA server refnum out"=w247:T77)  [unwired: 4 in]
          n70 = call "OPC Set Tag Name.vi"("error in (no error)"=w248, "name"=w237, "item node ID"=w246, "Refnum in"=w247) -> ("error out"=w253:errorcluster, "OPC Property cluster"=w244:T78)  [unwired: 6 in]
          n71 = call "OPC Set Tag Name.vi"("error in (no error)"=w248, "name"=w254, "item node ID"=w246, "Refnum in"=w247) -> ("error out"=w252:errorcluster, "OPC Property cluster"=w243:T78)  [unwired: 6 in]
          n72 = call "OPC Set Tag Name.vi"("error in (no error)"=w248, "name"=w255, "item node ID"=w246, "Refnum in"=w247) -> ("error out"=w251:errorcluster, "OPC Property cluster"=w242:T78)  [unwired: 6 in]
          n73 = call "OPC Set Tag Name.vi"("error in (no error)"=w248, "name"=w249, "item node ID"=w246, "Refnum in"=w247) -> ("error out"=w250:errorcluster, "OPC Property cluster"=w241:T78)  [unwired: 6 in]
          n74 = call "OPC Set Tag Name.vi"("error in (no error)"=w248, "name"=w245, "item node ID"=w246, "Refnum in"=w247) -> ("OPC Property cluster"=w240:T78)  [unwired: 6 in, 1 out]
          n75 = Build Array(w244, w243, w242, w241, w240) -> (w239:T3)
          n76 = Merge Errors(w253, w252, w251, w250) -> (w256:errorcluster)
        }
        n77 = for {
          tunnel: w41 -> [w113]
          tunnel: w60 -> [w112]
          tunnel: w61 -> [w111]
          tunnel: [w109] -> w55 mode=indexing
          tunnel: w59 -> [w110] mode=indexing
          tunnel: [w106] -> w62 mode=concatenating
          n78 = Unbundle By Name(w110) -> ("OPC UA Error"=w98:string, "Array of Names"=w101:string[])
          n79 = xnode "Match Regular Expression"("input string"=w98, "regular expression"="(.*):") -> ("submatch 1"=w97:string)  [unwired: 4 in, 5 out]
          n80 = call <vilib>:"Add Folder.vi"("error in (no error)"=w113, "folder name"=w97, "parent folder node ID"=w112, "OPC UA server refnum in"=w111) -> ("error out"=w105:errorcluster, "folder node ID"=w104:T1, "OPC UA server refnum out"=w103:T77)  [unwired: 4 in]
          n81 = for {
            tunnel: w105 -> [w235]
            tunnel: w104 -> [w234]
            tunnel: w103 -> [w233]
            tunnel: [w232] -> w102 mode=indexing
            tunnel: w101 -> [w231] mode=indexing
            tunnel: [w230] -> w100 mode=indexing
            n82 = call "OPC Set Tag Name.vi"("error in (no error)"=w235, "name"=w231, "item node ID"=w234, "Refnum in"=w233) -> ("error out"=w232:errorcluster, "OPC Property cluster"=w230:T78)  [unwired: 6 in]
          }
          n83 = call "OPC Set Tag Name.vi"("error in (no error)"=w105, "name"=w98, "item node ID"=w104, "Refnum in"=w103) -> ("error out"=w108:errorcluster, "OPC Property cluster"=w107:T78)  [unwired: 6 in]
          n84 = Build Array (concatenate)(w107, w100) -> (w106:T3)
          n85 = Merge Errors(w108, w102) -> (w109:errorcluster)
        }
        n86 = Merge Errors(w41, w49) -> (w48:errorcluster)
        n87 = Merge Errors(w41, w38) -> (w40:errorcluster)
        n88 = Merge Errors(w41, w47) -> (w46:errorcluster)
        n89 = Merge Errors(w41, w43) -> (w42:errorcluster)
        n90 = Merge Errors(w41, w45) -> (w44:errorcluster)
        n91 = Merge Errors(w41, w51) -> (w50:errorcluster)
        n92 = Merge Errors(w41, w53) -> (w52:errorcluster)
        n93 = Merge Errors(w41, w55) -> (w54:errorcluster)
        n94 = Merge Errors(w40, w42, w44, w46, w48, w50, w52, w54) -> (w75:errorcluster)
        n95 = call <vilib>:"Start.vi"("error in (no error)"=w75, "OPC UA server refnum in"=w58) -> ("error out"=w83:errorcluster, "OPC UA server refnum out"=w84:T77)  [unwired: 7 in, 1 out]
        n96 = Build Array (concatenate)(w69, w68, w67, w66, w65, w64, w63, w62) -> (w39:T3)
        "Array 4" <- w39
      }
      frame "Exit" {
        n97 = case shown="True" w1086 {
          tunnel: w1084 -> [w1094 w1107]
          tunnel: [w1094 w1096] -> w1091
          tunnel: w1090 -> [w1095 w1106]
          tunnel: [w1095 w1102] -> w1089
          tunnel: w1088 -> [w1093 w1103]
          tunnel: [w1093 w1103] -> w1085
          frame False {
          }
          frame True {
            # "7."
            n98 = flat-sequence {
              tunnel: w1106 -> [w1109]
              tunnel: w1107 -> [w1110]
              tunnel: [w1110] -> w1099
              tunnel: [w1109] -> w1098
              tunnel: [w1114] -> w1105
              tunnel: [w1113] -> w1104
              tunnel: w1099 -> [w1112]
              tunnel: w1098 -> [w1111]
              tunnel: w1105 -> [w1120]
              tunnel: w1104 -> [w1119]
              tunnel: w1103 -> [w1118]
              tunnel: [w1117] -> w1101
              tunnel: [w1116] -> w1100
              tunnel: [w1123] -> w1102
              tunnel: w1101 -> [w1122]
              tunnel: w1100 -> [w1123]
              tunnel: [w1121] -> w1097
              frame #0 {
                n99 = Wait (ms)(milliseconds to wait=u32 1) -> ()  [unwired: 1 out]
              }
              frame #1 {
                # "5."
                n100 = call <vilib>:"Stop.vi"("error in (no error)"=w1112, "OPC UA server refnum in"=w1111) -> ("error out"=w1113:errorcluster, "OPC UA server refnum out"=w1114:T77)  [unwired: 8 in]
              }
              frame #2 {
                # "6."
                n101 = call <vilib>:"Delete Node.vi"("error in (no error)"=w1119, "node ID"=w1118, "OPC UA server refnum in"=w1120) -> ("error out"=w1117:errorcluster, "OPC UA server refnum out"=w1116:T77)  [unwired: 7 in]
                n102 = Wait (ms)(milliseconds to wait=u32 100) -> ()  [unwired: 1 out]
              }
              frame #3 {
                n103 = call <vilib>:"Close.vi"("error in (no error)"=w1122, "OPC UA server refnum in"=w1123) -> ("error out"=w1121:errorcluster)  [unwired: 9 in]
              }
            }
            n104 = call <vilib>:"Clear Errors.vi"("error in (no error)"=w1097) -> ("error out"=w1096:errorcluster)  [unwired: 5 in, 1 out]
          }
        }
      }
      frame "Log" {
        n105 = call "Tag FGV.vi"("Operation"=Tag_FGV_Operation_Enum."Read All Tags", "error in (no error)"=w1133) -> ("Tag Names"=w1135:string[], "Tag Values"=w1127:dbl[], "error out"=w1132:errorcluster)  [unwired: 6 in, 5 out]
        "Tag Values" <- w1127
        "Tag Names" <- w1135
        n106 = for {
          tunnel: w1135 -> [w1146]
          tunnel: w1132 -> [w1141]
          tunnel: w1131 -> [w1147] mode=indexing
          tunnel: [w1147] -> w1130 mode=indexing
          tunnel: w1124 -> [w1142]
          tunnel: [w1140] -> w1129 mode=indexing
          tunnel: w1127 -> [w1139]
          tunnel: [w1137] -> w1126 mode=indexing
          n107 = Unbundle By Name(w1147) -> ("name"=w1145:string, "property node ID"=w1143:T1)
          n108 = Search 1D Array(1D array=w1146, element=w1145) -> (index of element=w1144:i32)  [unwired: 1 in]
          n109 = Index Array(array=w1139, index=w1144) -> (element=w1138:dbl)
          n110 = call-poly <vilib>:"Write.vi"("error in (no error)"=w1141, "value"=w1138, "node ID"=w1143, "OPC UA server refnum in"=w1142) -> ("error out"=w1140:errorcluster, "status"=w1137:T17)  [unwired: 5 in, 1 out]
        }
        "Array" <- w1130
        "Array 2" <- w1126
        n111 = Merge Errors(w1129) -> (w1128:errorcluster)
        "OPC UA server refnum out" <- w1124
      }
    }
    "OPC UA server refnum out 3" <- w24
    "Array 3" <- w19
  }
